vi "Indentify Prema.vi"(8 "error in":errorcluster, 11 "VISA resource name":refnum<visa-resource-name>) -> (0 "error out":errorcluster, 1 "Instrument":T1, 2 "Is Prema?":bool, 3 "VISA resource name out":refnum<visa-resource-name>)   [LabVIEW 2021]
uses:
  Device/Device type.ctl
panel:
  out "read buffer":string
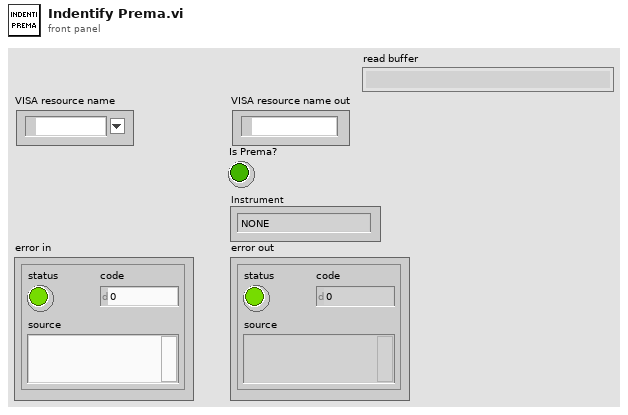
[diagram p1: front panel]
types:
  T1 = typedef "Device type.ctl" = enum16{"NONE", "Neocera 21", "LakeShore 335", "LakeShore 336", "LakeShore 340", "LkShr 340 chA&B", "LakeShore 370", "SRS 850", "SRS 830", "LR 700", "EG&G 5302", "EG&G 7260", "EG&G 7265", "EG&G 7280", "AH 2500", "AH 2550", "AH 2700", "Keithley meter", "Keithley electrometer", "Keithley 182", "HP 5385", "HP 53181", "HP 53132", "ITC503", "IPS120", "Oxford Mercury IPS", "Oxford PS", "Test", "DC Facility Magnet", "Cryomagnetics PS", "Keithley 2400", "Keithley current source", "Cryo-Con 22C", "HP87NN", "HP4395A", "Agilent 34410A", "Arduino TC", "Cryo-Con 54", "Fluke 1586A", "Prema"}
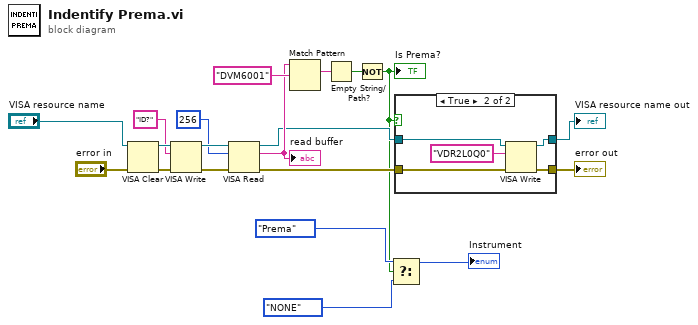
[diagram p0: block diagram]
diagram:
  n1 = VISA Clear(VISA resource name="VISA resource name", error in (no error)="error in") -> (VISA resource name out=w20:refnum<visa-resource-name>, error out=w19:errorcluster)
  n2 = VISA Write(VISA resource name=w20, write buffer="ID?", error in (no error)=w19) -> (VISA resource name out=w17:refnum<visa-resource-name>, error out=w16:errorcluster)  [unwired: 1 out]
  n3 = VISA Read(VISA resource name=w17, byte count=u32 256, error in (no error)=w16) -> (VISA resource name out=w7:refnum<visa-resource-name>, read buffer=w9:string, error out=w8:errorcluster)  [unwired: 1 out]
  "read buffer" <- w9
  n4 = Match Pattern(string=w9, regular expression="DVM6001") -> (match substring=w11:string)  [unwired: 1 in, 3 out]
  n5 = Empty String/Path?(string/path=w11) -> (empty?=w10:bool)
  n6 = Not(x=w10) -> (.not. x?=w1:bool)
  "Is Prema?" <- w1
  n7 = Select(t=Device_type."Prema" ("Instrument"), s=w1, f=Device_type."NONE" ("s? t:f")) -> (s? t:f=→"Instrument":T1)
  n8 = case shown="True" w1 {
    tunnel: w8 -> [w22 w27]
    tunnel: w7 -> [w21 w26]
    tunnel: [w22 w24] -> w6
    tunnel: [w21 w23] -> w5
    frame False {
    }
    frame True {
      n9 = VISA Write(VISA resource name=w26, write buffer="VDR2L0Q0", error in (no error)=w27) -> (VISA resource name out=w23:refnum<visa-resource-name>, error out=w24:errorcluster)  [unwired: 1 out]
    }
  }
  "error out" <- w6
  "VISA resource name out" <- w5
